vi "CollisionAvoidance.vi"(8 "error in":errorcluster) -> (0 "error out":errorcluster)   [LabVIEW 2009, in "Main.lvlib"]
doc: "Collision Avoidance algorithm. Check if there is an obstacle in front and aborts position control if any."
uses:
  Main.lvlib
  Drive.lvlib
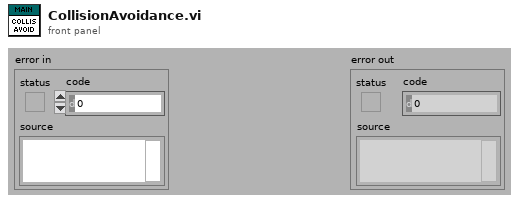
[diagram p1: front panel]
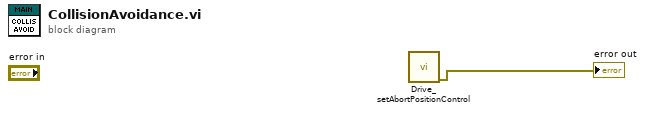
[diagram p0: block diagram]
diagram:
  n1 = call "Drive_setAbortPositionControl.vi"() -> ("error out"=→"error out":errorcluster)  [unwired: 11 in]
